vi "post build add to repo.vi"() -> ()   [LabVIEW 2013]
uses:
  <vilib>/JKI/VIPM API/VIPM API_vipm_api.lvlib
panel:
  out "error out":errorcluster
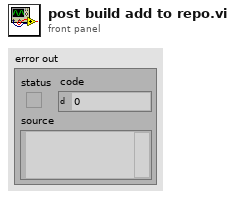
[diagram p1: front panel]
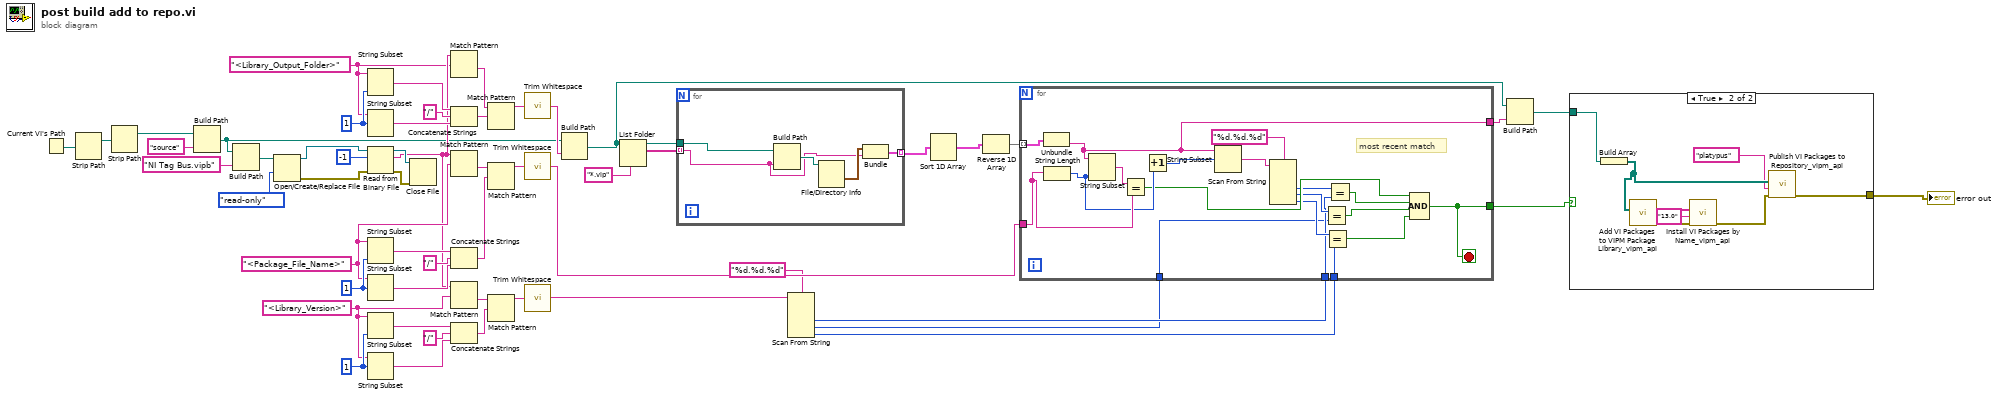
[diagram p0: block diagram]
diagram:
  w21 = "<Library_Output_Folder>" ("regular expression")
  w27 = 1 ("length (rest)")
  w31 = "<Library_Version>" ("regular expression")
  w33 = 1 ("length (rest)")
  w44 = 1 ("length (rest)")
  w43 = "<Package_File_Name>" ("regular expression")
  n1 = Current VI's Path() -> (path=w56:path)
  n2 = Strip Path(path=w56) -> (stripped path=w55:path)  [unwired: 1 out]
  n3 = Strip Path(path=w55) -> (stripped path=w53:path)  [unwired: 1 out]
  n4 = Build Path(base path=w53, name or relative path="source") -> (appended path=w18:path)
  n5 = Build Path(base path=w18, name or relative path="NI Tag Bus.vipb") -> (appended path=w20:path)
  n6 = Open/Create/Replace File(file path (use dialog)=w20, access (0:read/write)=enum16{"read/write", "read-only", "write-only"}."read-only") -> (refnum out=w50:refnum<file>, error out=w49:errorcluster)  [unwired: 4 in, 1 out]
  n7 = String Subset(string=w21, length (rest)=w27) -> (substring=w26:string)  [unwired: 1 in]
  n8 = String Subset(string=w21, offset (0)=w27) -> (substring=w25:string)  [unwired: 1 in]
  n9 = Read from Binary File(8:w49, 10:-1 ("count (1)"), 11:w50) -> (0:w46:errorcluster, 2:w22:string, 3:w47:refnum<file>)  [unwired: 3 in, 1 out]
  n10 = String Subset(string=w43, length (rest)=w44) -> (substring=w42:string)  [unwired: 1 in]
  n11 = String Subset(string=w43, offset (0)=w44) -> (substring=w41:string)  [unwired: 1 in]
  n12 = String Subset(string=w31, length (rest)=w33) -> (substring=w34:string)  [unwired: 1 in]
  n13 = String Subset(string=w31, offset (0)=w33) -> (substring=w35:string)  [unwired: 1 in]
  n14 = Close File(refnum=w47, error in=w46) -> ()  [unwired: 2 out]
  n15 = Match Pattern(string=w22, regular expression=w21) -> (after substring=w28:string)  [unwired: 1 in, 3 out]
  n16 = Concatenate Strings(w26, "/" ("string"), w25) -> (w23:string)
  n17 = Match Pattern(string=w22, regular expression=w43) -> (after substring=w45:string)  [unwired: 1 in, 3 out]
  n18 = Concatenate Strings(w42, "/" ("string"), w41) -> (w39:string)
  n19 = Match Pattern(string=w22, regular expression=w31) -> (after substring=w32:string)  [unwired: 1 in, 3 out]
  n20 = Concatenate Strings(w34, "/" ("string"), w35) -> (w37:string)
  n21 = Match Pattern(string=w28, regular expression=w23) -> (before substring=w29:string)  [unwired: 1 in, 3 out]
  n22 = Match Pattern(string=w45, regular expression=w39) -> (before substring=w38:string)  [unwired: 1 in, 3 out]
  n23 = Match Pattern(string=w32, regular expression=w37) -> (before substring=w30:string)  [unwired: 1 in, 3 out]
  n24 = call <vilib>:"Trim Whitespace.vi"("string"=w29) -> ("trimmed string"=w19:string)  [unwired: 1 in]
  n25 = call <vilib>:"Trim Whitespace.vi"("string"=w38) -> ("trimmed string"=w11:string)  [unwired: 1 in]
  n26 = call <vilib>:"Trim Whitespace.vi"("string"=w30) -> ("trimmed string"=w9:string)  [unwired: 1 in]
  n27 = Build Path(base path=w18, name or relative path=w19) -> (appended path=w4:path)
  n28 = List Folder(path=w4, pattern="*.vip") -> (path out=w16:path, filenames=w15:string[])  [unwired: 2 in, 2 out]
  n29 = for {
    tunnel: w16 -> [w61]
    tunnel: w15 -> [w58] mode=indexing
    tunnel: [w57] -> w14 mode=indexing
    n30 = Build Path(base path=w61, name or relative path=w58) -> (appended path=w60:path)
    n31 = File/Directory Info(path=w60) -> (last mod=w59:timestamp)  [unwired: 1 in, 6 out]
    n32 = Bundle("last mod"=w59, w58) -> (w57:cluster{"last mod":timestamp, string})  [unwired: 1 in]
  }
  n33 = Scan From String(format string="%d.%d.%d", input string=w9) -> (output 1=w8:i32, output 2=w7:i32, output 3=w6:i32)  [unwired: 5 in, 3 out]
  n34 = Sort 1D Array(array=w14) -> (sorted array=w13:cluster{"last mod":timestamp, string}[])
  n35 = Reverse 1D Array(array=w13) -> (reversed array=w12:cluster{"last mod":timestamp, string}[])
  n36 = for {
    tunnel: w12 -> [w80] mode=indexing
    tunnel: w11 -> [w78]
    tunnel: w8 -> [w66]
    tunnel: w7 -> [w65]
    tunnel: w6 -> [w64]
    tunnel: [w63] -> w5
    tunnel: [w62] -> w3
    stop <- w62 stop-if-true
    # "most recent match"
    n37 = Unbundle(w80) -> (w63:string)  [unwired: 1 out]
    n38 = String Length(string=w78) -> (length=w76:i32)
    n39 = String Subset(string=w63, length (rest)=w76) -> (substring=w79:string)  [unwired: 1 in]
    n40 = Equal?(x=w79, y=w78) -> (x = y?=w73:bool)
    n41 = Increment(x=w76) -> (x+1=w77:i32)
    n42 = String Subset(string=w63, offset (0)=w77) -> (substring=w75:string)  [unwired: 1 in]
    n43 = Scan From String(format string="%d.%d.%d", input string=w75) -> (output 1=w69:i32, output 2=w68:i32, output 3=w67:i32)  [unwired: 5 in, 3 out]
    n44 = Equal?(x=w68, y=w65) -> (x = y?=w71:bool)
    n45 = Equal?(x=w67, y=w64) -> (x = y?=w70:bool)
    n46 = Equal?(x=w69, y=w66) -> (x = y?=w72:bool)
    n47 = Compound Arithmetic op=AND(w73, w72, w71, w70) -> (w62:bool)
  }
  n48 = Build Path(base path=w4, name or relative path=w5) -> (appended path=w2:path)
  n49 = case shown="True" w3 {
    tunnel: w2 -> [_ w88]
    tunnel: [_ w82] -> w1
    frame False {
    }
    frame True {
      n50 = Build Array(w88) -> (w87:path[])
      n51 = call <vilib>:"Add VI Packages to VIPM Package Library_vipm_api.vi"("Packages to add to VIPM Library (vipc,vip,ogp)"=w87) -> ("error out"=w86:errorcluster, "Package Names Added"=w85:string[])  [unwired: 9 in]
      n52 = call <vilib>:"Install VI Packages by Name_vipm_api.vi"("error in (no error)"=w86, "LabVIEW Version"="13.0", "Package Names to Install []"=w85) -> ("error out"=w83:errorcluster)  [unwired: 8 in]
      n53 = call <vilib>:"Publish VI Packages to Repository_vipm_api.vi"("error in (no error)"=w83, "Repository Name"="platypus", "Packages to publish to Repository Library (vip,ogp)"=w87) -> ("error out"=w82:errorcluster)  [unwired: 7 in, 1 out]
    }
  }
  "error out" <- w1
